vi "LoadHeader.vi"(4 "Path":path) -> (0 "error out":errorcluster)   [LabVIEW 2009]
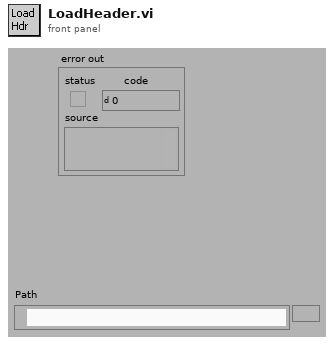
[diagram p1: front panel]
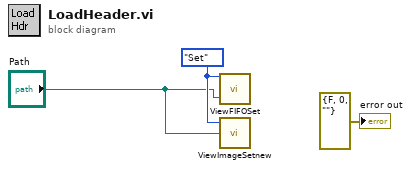
[diagram p0: block diagram]
diagram:
  w2 = enum16{"Display", "change", "Get", "Set"}."Set" ("Enum")
  n1 = call "ViewFIFOSet.vi"("Path"="Path", "Enum"=w2) -> ()  [unwired: 1 out]
  n2 = call "ViewImageSetnew.vi"("Path"="Path", "action"=w2) -> ()  [unwired: 1 in, 1 out]
  "error out" <- errorcluster {"status"=FALSE, "code"=0, "source"=""} ("error out")
